vi "ClearHeaders.vi"(8 "error in (no error)":errorcluster, 11 "Refnum in":T1) -> (0 "error out":errorcluster, 3 "Refnum out":T1)   [LabVIEW 2016]
uses:
  <vilib>/httpClient/LabVIEWHTTPClient.lvlib
  <vilib>/httpClient/ClientHandle.ctl
panel:
  out "subarray":string[](array[string])
  out "headers":string
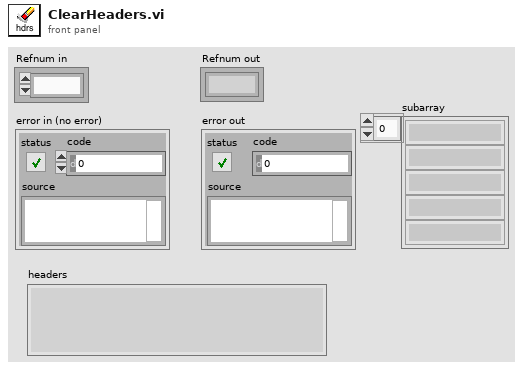
[diagram p1: front panel]
types:
  T1 = typedef "LabVIEWHTTPClient.lvlib/ClientHandle.ctl" = refnum<k1>
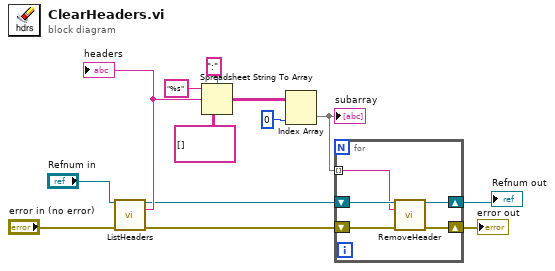
[diagram p0: block diagram]
diagram:
  n1 = call <vilib>:"ListHeaders.vi"("client handle"="Refnum in", "error in (no error)"="error in (no error)") -> ("client handle out"=w5:T1, "headers"=w11:string, "error out"=w3:errorcluster)  [unwired: 11 in]
  "headers" <- w11
  n2 = Spreadsheet String To Array(delimiter (Tab)=":", format string="%s", spreadsheet string=w11, array type (2D Dbl)=string[][] []) -> (array=w7:string[][])
  n3 = Index Array(array=w7, index (col)=0 ("disabled index (col)")) -> (element=w4:string[])  [unwired: 1 in]
  "subarray" <- w4
  n4 = for {
    tunnel: w4 -> [w17] mode=indexing
    shift-right: [w15] -> w2
    shift-left: w5 -> [w18]
    shift-right: [w14] -> w1
    shift-left: w3 -> [w16]
    n5 = call <vilib>:"RemoveHeader.vi"("client handle"=w18, "header"=w17, "error in (no error)"=w16) -> ("client handle out"=w15:T1, "error out"=w14:errorcluster)  [unwired: 11 in]
  }
  "Refnum out" <- w2
  "error out" <- w1
